vi "Thumbstick Config.vi"(0 "Arduino Resource":T1={"VISA resource"="", "Board Type"=enum."Uno", "Connection Type"=enum."USB / Serial", "Bytes Per Packet (15)"=15}, 5 "Horizontal Axis AI Pin":u8, 7 "Vertical Axis AI Pin":u8, 9 "Select DI Pin":u8, 11 "error in":errorcluster) -> (4 "Arduino Resource":T1={"VISA resource"="", "Board Type"=enum."Uno", "Connection Type"=enum."USB / Serial", "Bytes Per Packet (15)"=15}, 8 "Thumbstick Data":T3, 15 "error out":errorcluster)   [LabVIEW 2011, in "LabVIEW Interface for Arduino.lvlib"]
doc: "Configure two Arduino analog inputs and one Arduino digital input for use with a thumb stick."
uses:
  <vilib>/LabVIEW Interface for Arduino/LabVIEW Interface for Arduino.lvlib
  <vilib>/LabVIEW Interface for Arduino/Private/Type Defs/Arduino Resource.ctl
  <vilib>/LabVIEW Interface for Arduino/Private/Type Defs/Board Type.ctl
  <vilib>/LabVIEW Interface for Arduino/Private/Type Defs/Pin Mode.ctl
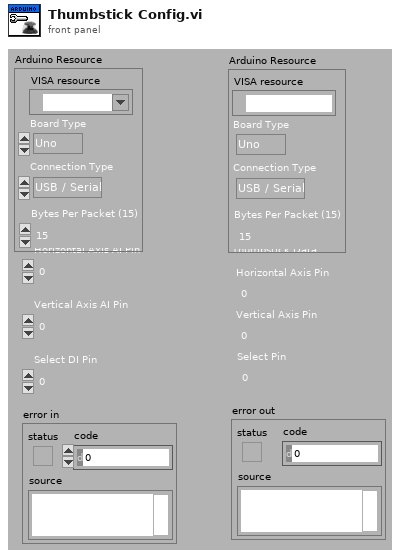
[diagram p1: front panel]
types:
  T1 = typedef "LabVIEW Interface for Arduino.lvlib/Arduino Resource.ctl" = cluster{"VISA resource":refnum<visa-resource-name>, "Board Type":T2, "Connection Type":enum8{"USB / Serial"}, "Bytes Per Packet (15)":u8}
  T2 = typedef "LabVIEW Interface for Arduino.lvlib/Board Type.ctl" = enum16{"Uno", "Dimuelanove w/Atmega 328", "Mega 2560"}
  T3 = cluster{"Horizontal Axis Pin":dbl, "Vertical Axis Pin":dbl, "Select Pin":dbl}
  T4 = typedef "LabVIEW Interface for Arduino.lvlib/Pin Mode.ctl" = enum8{"Input", "Output"}
  T5 = cluster{"Horizontal Axis AI Pin":u8, "Vertical Axis AI Pin":u8, "Select DI Pin":u8}
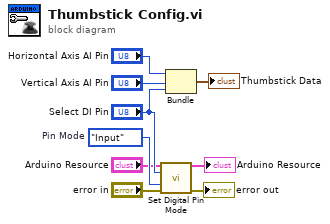
[diagram p0: block diagram]
diagram:
  w7 = Pin_Mode."Input"  # Pin Mode
  n1 = call <vilib>:"Set Digital Pin Mode.vi"("Arduino Resource"="Arduino Resource", "Digital I/O Pin"="Select DI Pin", "Pin Mode (Input)"=w7, "error in"="error in") -> ("Arduino Resource"=→"Arduino Resource":T1, "error out"=→"error out":errorcluster)  [unwired: 10 in]
  n2 = Bundle("Horizontal Axis AI Pin"="Horizontal Axis AI Pin", "Vertical Axis AI Pin"="Vertical Axis AI Pin", "Select DI Pin"="Select DI Pin") -> (→"Thumbstick Data":T5)  [unwired: 1 in]
